vi "encoder.vi"() -> (2 "Mes Pos (mm)":dbl[](array[numeric]), 3 "RPM":dbl[](array[knob]) scale=-200.0..200.0)   [LabVIEW 2021]
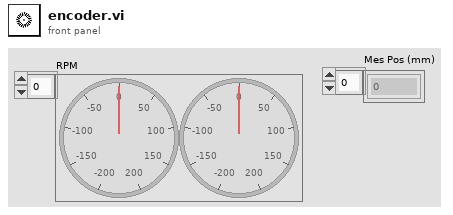
[diagram p1: front panel]
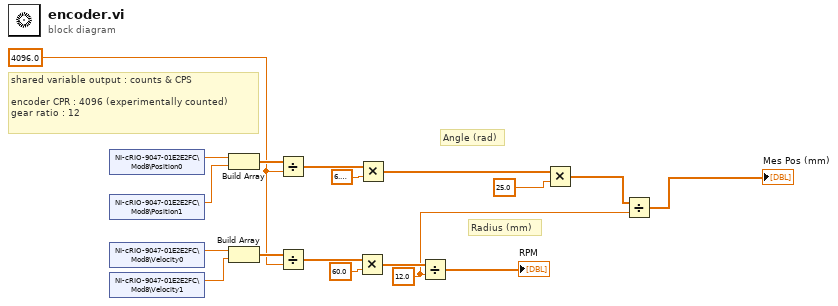
[diagram p0: block diagram]
diagram:
  w1 = 12.0 ("y")
  w6 = 4096.0 ("y")
  # "Radius (mm)"
  # "Angle (rad)"
  # "shared variable output : counts & CPS\n\nencoder CPR : 4096 (experimentally counted)\ngear ratio : 12"
  n1 = shared-variable "NI-cRIO-9047-01E2E2FC\\Mod8\\Position0"() -> (w11:dbl)  [unwired: 1 in, 1 out]
  n2 = shared-variable "NI-cRIO-9047-01E2E2FC\\Mod8\\Position1"() -> (w10:dbl)  [unwired: 1 in, 1 out]
  n3 = shared-variable "NI-cRIO-9047-01E2E2FC\\Mod8\\Velocity0"() -> (w15:dbl)  [unwired: 1 in, 1 out]
  n4 = shared-variable "NI-cRIO-9047-01E2E2FC\\Mod8\\Velocity1"() -> (w14:dbl)  [unwired: 1 in, 1 out]
  n5 = Build Array(w11, w10) -> (w12:dbl[])
  n6 = Build Array(w15, w14) -> (w13:dbl[])
  n7 = Divide(x=w12, y=w6) -> (x/y=w8:dbl[])
  n8 = Divide(x=w13, y=w6) -> (x/y=w18:dbl[])
  n9 = Multiply(x=w18, y=60.0) -> (x*y=w16:dbl[])
  n10 = Multiply(x=w8, y=6.283185307179586) -> (x*y=w5:dbl[])
  n11 = Divide(x=w16, y=w1) -> (x/y=→"RPM":dbl[])
  n12 = Multiply(x=w5, y=25.0) -> (x*y=w3:dbl[])
  n13 = Divide(x=w3, y=w1) -> (x/y=→"Mes Pos (mm)":dbl[])
